vi "StopGui.vi"(0 "reference in":refnum<class "RemoteControl.lvclass">, 2 "ms timeout (-1)":i32=-1, 5 "error in (no error)":errorcluster) -> (14 "reference out":refnum<class "RemoteControl.lvclass">, 19 "error out":errorcluster)   [LabVIEW 2020, in "RemoteControl.lvclass"]
uses:
  RemoteControl.lvclass
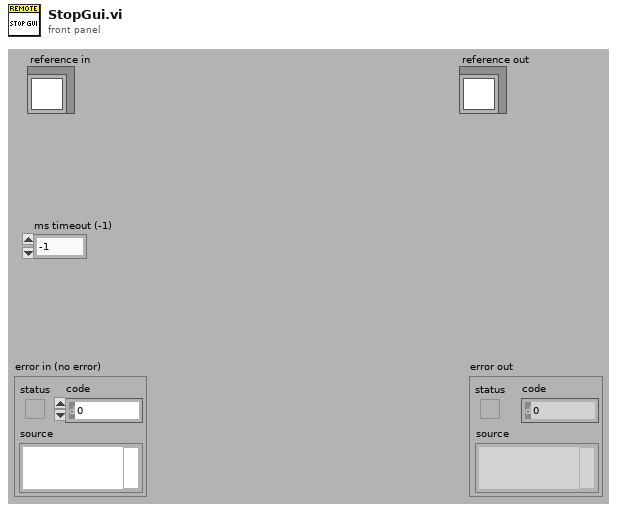
[diagram p1: front panel]
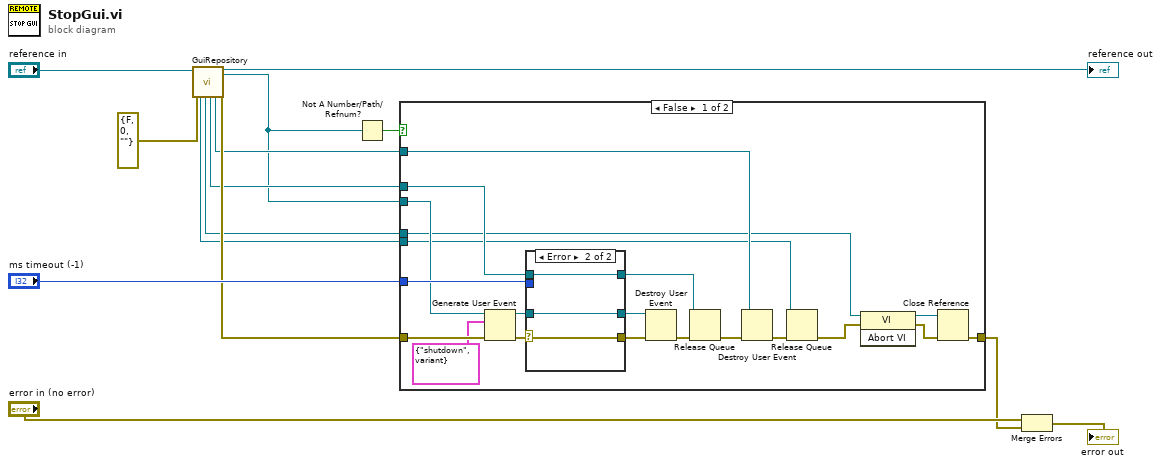
[diagram p0: block diagram]
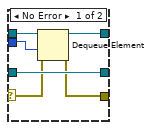
[diagram p2: hidden frame]
diagram:
  n1 = call "GuiRepository.vi"("reference in"="reference in", "error in (no error)"=errorcluster {"status"=FALSE, "code"=0, "source"=""}) -> ("QueueFromProcess"=w1:refnum<queue>, "ProcessViRef"=w5:refnum<vi>, "ProcessSyncQueue"=w7:refnum<queue>, "EventFromProcess"=w6:refnum<user-event>, "reference out"=→"reference out":refnum<class "RemoteControl.lvclass">, "EventsToProcess"=w3:refnum<user-event>, "error out"=w8:errorcluster)  [unwired: 10 in, 1 out]
  n2 = Not A Number/Path/Refnum?(number/path/refnum=w3) -> (NaN/Path/Refnum?=w2:bool)
  n3 = case shown="False" w2 {
    tunnel: w7 -> [w34 _]
    tunnel: w8 -> [w26 w44]
    tunnel: [w30 w44] -> w12
    tunnel: w3 -> [w25 _]
    tunnel: "ms timeout (-1)" -> [w29 _]
    tunnel: w6 -> [w27 _]
    tunnel: w5 -> [w23 _]
    tunnel: w1 -> [w19 _]
    frame False {
      n4 = Generate User Event(user event=w25, event data cluster=cluster{"Command":string, "Data":variant} {"Command"="shutdown", "Data"=variant} ("event data"), error in=w26) -> (user event out=w33:refnum<user-event>, error out=w28:errorcluster)  [unwired: 1 in]
      n5 = case shown="Error" w28 {
        tunnel: [w38 w43] -> w32
        tunnel: w34 -> [w37 w41]
        tunnel: [w40 w42] -> w31
        tunnel: w33 -> [w40 w42]
        tunnel: w29 -> [w36 _]
        selector: w28 -> [w39 w43]
        tunnel: [w35 w41] -> w15
        frame No Error {
          n6 = Dequeue Element(queue=w37, timeout in ms (-1)=w36, error in (no error)=w39) -> (queue out=w35:refnum<queue>, error out=w38:errorcluster)  [unwired: 2 out]
        }
        frame Error {
        }
      }
      n7 = Destroy User Event(user event=w31, error in=w32) -> (error out=w17:errorcluster)
      n8 = Release Queue(queue=w15, error in (no error)=w17) -> (error out=w16:errorcluster)  [unwired: 1 in, 2 out]
      n9 = Destroy User Event(user event=w27, error in=w16) -> (error out=w20:errorcluster)
      n10 = Release Queue(queue=w19, error in (no error)=w20) -> (error out=w18:errorcluster)  [unwired: 1 in, 2 out]
      n11 = invoke class="VI" method="Abort VI"(reference=w23, error in=w18) -> (reference out=w22:refnum<vi>, error out=w21:errorcluster)  [unwired: 1 in, 1 out]
      n12 = Close Reference(reference=w22, error in (no error)=w21) -> (error out=w30:errorcluster)
    }
    frame True {
    }
  }
  n13 = Merge Errors("error in (no error)", w12) -> (→"error out":errorcluster)
